vi "Obtain Status.vi"(8 "Error In":errorcluster, 11 "Application In":refnum<class "Application.lvclass">) -> (0 "Error Out":errorcluster, 1 "Status":string, 2 "Page":T1(ring), 3 "Application Out":refnum<class "Application.lvclass">)   [LabVIEW 2019, in "Application.lvclass"]
doc: "The VI obtains the current page to be redirected and the status to be displayed."
uses:
  Application.lvclass
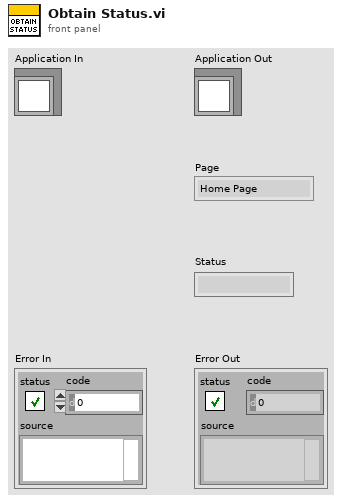
[diagram p1: front panel]
types:
  T1 = enum32{"Home Page", "Mode Page", "Configuration Page", "Input Page", "Result Page"}
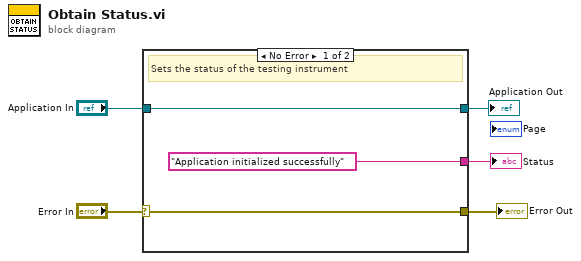
[diagram p0: block diagram]
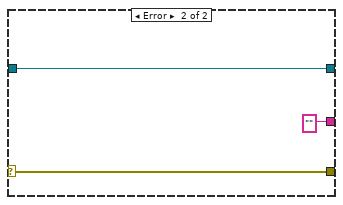
[diagram p2: hidden frame]
diagram:
  n1 = case shown="No Error" "Error In" {
    selector: "Error In" -> [w7 w11]
    tunnel: [w7 w11] -> w4
    tunnel: [w8 w10] -> w2
    tunnel: "Application In" -> [w8 w10]
    tunnel: ["Application initialized successfully" ("String") "" ("String")] -> w1
    frame No Error {
      # "Sets the status of the testing instrument"
    }
    frame Error {
    }
  }
  "Error Out" <- w4
  "Application Out" <- w2
  "Status" <- w1
